vi "PH_OceanOpticsSpectrometer.get data to modify.vi"(0 "i ref in":refnum<vi>, 3 "ms timeout (10000)":i32=10000, 5 "error in (no error)":errorcluster) -> (14 "i ref out":refnum<vi>, 16 "i attribute":T1={"GUI Refs"={"Delete"=refnum, "Spectrum"=refnum, "Display Width"=refnum, "Display Center"=refnum, "Save"=refnum, "Integration time"=refnum, "center wavelength"=refnum, "width"=refnum, "Wanted Trigger Mode"=refnum, "Current Trigger Mode"=refnum, "Trigger Info"=refnum, "Model"=refnum, "Driver"=refnum, "Firmware"=refnum}, "Display"={"Width"=50.0, "Center"=1054.0}, "VISA resource name"="N/A", "Integration time [ms]"={"Current Value"=100, "Wanted Value"=100}, "Trigger"={"Current value"=enum."Normal", "Wanted value"=enum."Normal"}, "Default VISA Timeout"=0, "Last Data"={"Wavelength Bins"=[], "Spectrum by Pixels"=[]}} {"Integration time [ms]"."Wanted Value" min=1 max=500 step=1; "Integration time [ms]"."Current Value" min=1 max=500 step=1}, 17 "timed out":bool, 19 "error out":errorcluster)   [LabVIEW 2014, in "PH_OceanOpticsSpectrometer.lvlib"]
doc: "Reads the attribute data of the object after the access to the data has been locked by the \"acquire\" method. If the attribute data has been locked already, this methods waits until the attribute data is unlocked or there is a timeout.\n\nThe attribute data must be unlocked using the methods \"release\" or \"set modified data\".\n\nLicense Agreement for this software:\n\nCopyright (C)\nGesellschaft für Schwerionenforschung, GSI\nPlanckstr. 1\n64291 Darmstadt\nGermany\n\nContact: D.Beck@gsi.de \n\nThis program is free software; you can redistribute it and/or modify it under the terms of the GNU General Public License as published by the Free Software Foundation; either version 2 of the license, or (at your option) any later version.\n\nThis program is distributed in the hope that it will be useful, but WITHOUT ANY WARRANTY; without even the implied warranty of MERCHANTABILITY or FITNESS FOR A PARTICULAR PURPOSE. See the GNU General License for more details (http://www.gnu.org).\n\nGesellschaft für Schwerionenforschung, GSI\nPlanckstr. 1, 64291 Darmstadt, Germany\nFor all questions and ideas contact: M.Richter@gsi.de, H.Brand@gsi.de or D.Beck@gsi.de.\nLast update: 17-JUN-2004"
uses:
  PH_OceanOpticsSpectrometer.lvlib
  PH_OceanOpticsSpectrometer.i attribute.ctl
  PH_OceanOpticsSpectrometer.Trigger.ctl
  CS_Core/CSObj/CSObj.lvlib
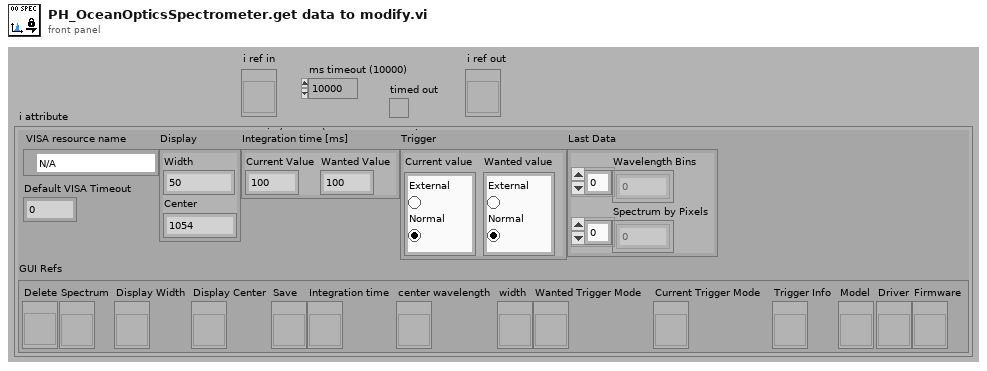
[diagram p1: front panel]
types:
  T1 = typedef "PH_OceanOpticsSpectrometer.lvlib/PH_OceanOpticsSpectrometer.i attribute.ctl" = cluster{"GUI Refs":cluster{"Delete":refnum<vi>, "Spectrum":refnum<vi>, "Display Width":refnum<vi>, "Display Center":refnum<vi>, "Save":refnum<vi>, "Integration time":refnum<vi>, "center wavelength":refnum<vi>, "width":refnum<vi>, "Wanted Trigger Mode":refnum<vi>, "Current Trigger Mode":refnum<vi>, "Trigger Info":refnum<vi>, "Model":refnum<vi>, "Driver":refnum<vi>, "Firmware":refnum<vi>}, "Display":cluster{"Width":dbl, "Center":dbl}, "VISA resource name":refnum<visa-resource-name>, "Integration time [ms]":cluster{"Current Value":u16, "Wanted Value":u16}, "Trigger":cluster{"Current value":T2, "Wanted value":T2}, "Default VISA Timeout":u32, "Last Data":cluster{"Wavelength Bins":dbl[], "Spectrum by Pixels":dbl[]}}
  T2 = typedef "PH_OceanOpticsSpectrometer.lvlib/PH_OceanOpticsSpectrometer.Trigger.ctl" = enum32{"External", "Normal"}
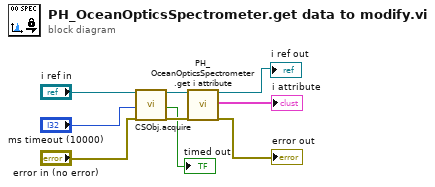
[diagram p0: block diagram]
diagram:
  n1 = call "CSObj.acquire.vi"("i ref in"="i ref in", "ms timeout (10000)"="ms timeout (10000)", "error in (no error)"="error in (no error)") -> ("i ref out"=w8:refnum<vi>, "timed out"=→"timed out":bool, "error out"=w5:errorcluster)  [unwired: 14 in]
  n2 = call "PH_OceanOpticsSpectrometer.get i attribute.vi"("i ref in"=w8, "error in (no error)"=w5) -> ("i ref out"=→"i ref out":refnum<vi>, "i attribute"=→"i attribute":T1, "error out"=→"error out":errorcluster)  [unwired: 15 in]
